vi "roboRIO v1.0 Write DIO.vi"(8 "error in (no error)":errorcluster, 9 "bool Value List":bool[](array[boolean]), 10 "Channel List":T3, 11 "myRIO Ref In":T1) -> (0 "error out":errorcluster, 3 "myRIO Ref Out":T1)   [LabVIEW 2021]
uses:
  <vilib>/myRIO/Common/Instrument Driver Framework/myRIO v1.0/DIO/typedefs/DIO Channels List.ctl
  <vilib>/myRIO/Common/Instrument Driver Framework/myRIO v1.0/DIO/typedefs/DIO Channels Enum.ctl
  <vilib>/myRIO/Common/Instrument Driver Framework/Utilities/typedefs/myRIO v1.0 Reference.ctl
  <vilib>/myRIO/Common/Instrument Driver Framework/Utilities/typedefs/Generic FPGA Reference.ctl
  <vilib>/myRIO/Common/Instrument Driver Framework/roboRIO v1.0/DIO/typedefs/roboRIO DIO FPGA Reference.ctl
  <vilib>/myRIO/Common/Instrument Driver Framework/roboRIO v1.0/DIO/typedefs/roboRIO DIO Bank Enum.ctl
  <vilib>/rvi/errors/niLvFpgaAdjustHostInterfaceError.vi
  <vilib>/rvi/interface/nirviReadWriteControl/nirviReadWriteControl.xnode
  <vilib>/rvi/interface/Simulation/niFpgaSimulationCallBeginRW.vi
  NiFpgaLv.dll
panel:
  # "This VI writes boolean values to a user specified a list of DIO channels on the myRIO v1.0 hardware. The value is input as a boolean value. Please see Block Diagram for details."
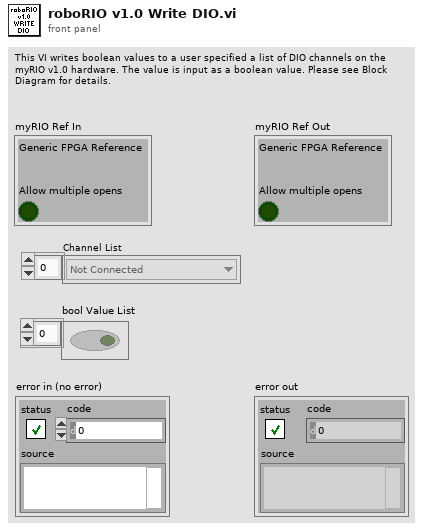
[diagram p1: front panel]
types:
  T1 = typedef "myRIO v1.0 Reference.ctl" = cluster{"Generic FPGA Reference":T2, "Allow multiple opens":bool}
  T2 = typedef "Generic FPGA Reference.ctl" = refnum<k20>
  T3 = typedef "DIO Channels List.ctl" = T4[]
  T4 = typedef "DIO Channels Enum.ctl" = enum16{"Not Connected", "C/DIO0", "C/DIO1", "C/DIO2", "C/DIO3", "C/DIO4", "C/DIO5", "C/DIO6", "C/DIO7", "A/DIO0", "A/DIO1", "A/DIO2", "A/DIO3", "A/DIO4", "A/DIO5", "A/DIO6", "A/DIO7", "A/DIO8", "A/DIO9", "A/DIO10", "A/DIO11", "A/DIO12", "A/DIO13", "A/DIO14", "A/DIO15", "A/DIO16", "A/DIO17", "A/DIO18", "A/DIO19", "B/DIO0", "B/DIO1", "B/DIO2", "B/DIO3", "B/DIO4", "B/DIO5", "B/DIO6", "B/DIO7", "B/DIO8", "B/DIO9", "B/DIO10", "B/DIO11", "B/DIO12", "B/DIO13", "B/DIO14", "B/DIO15", "B/DIO16", "B/DIO17", "B/DIO18", "B/DIO19", "LED0", "LED1", "LED2", "LED3", "Button0", "DIO/DIO0", "DIO/DIO1", "DIO/DIO2", "DIO/DIO3", "DIO/DIO4", "DIO/DIO5", "DIO/DIO6", "DIO/DIO7", "DIO/DIO8", "DIO/DIO9", "SPI/CS0", "SPI/CS1", "SPI/CS2", "SPI/CS3", "LED RADIO (Green)", "LED RADIO (Red)", "LED COMM (Green)", "LED COMM (Red)", "LED MODE (Green)", "LED MODE (Red)"}
  T5 = typedef "roboRIO DIO Bank Enum.ctl" = enum32{"None", "B/DIO7:0", "B/DIO15:8", "DIO/DIO7:0", "DIO/DIO9:8", "SPI/CS3:0", "LED", "Button0"}
  T6 = typedef "roboRIO DIO FPGA Reference.ctl" = refnum<k20>
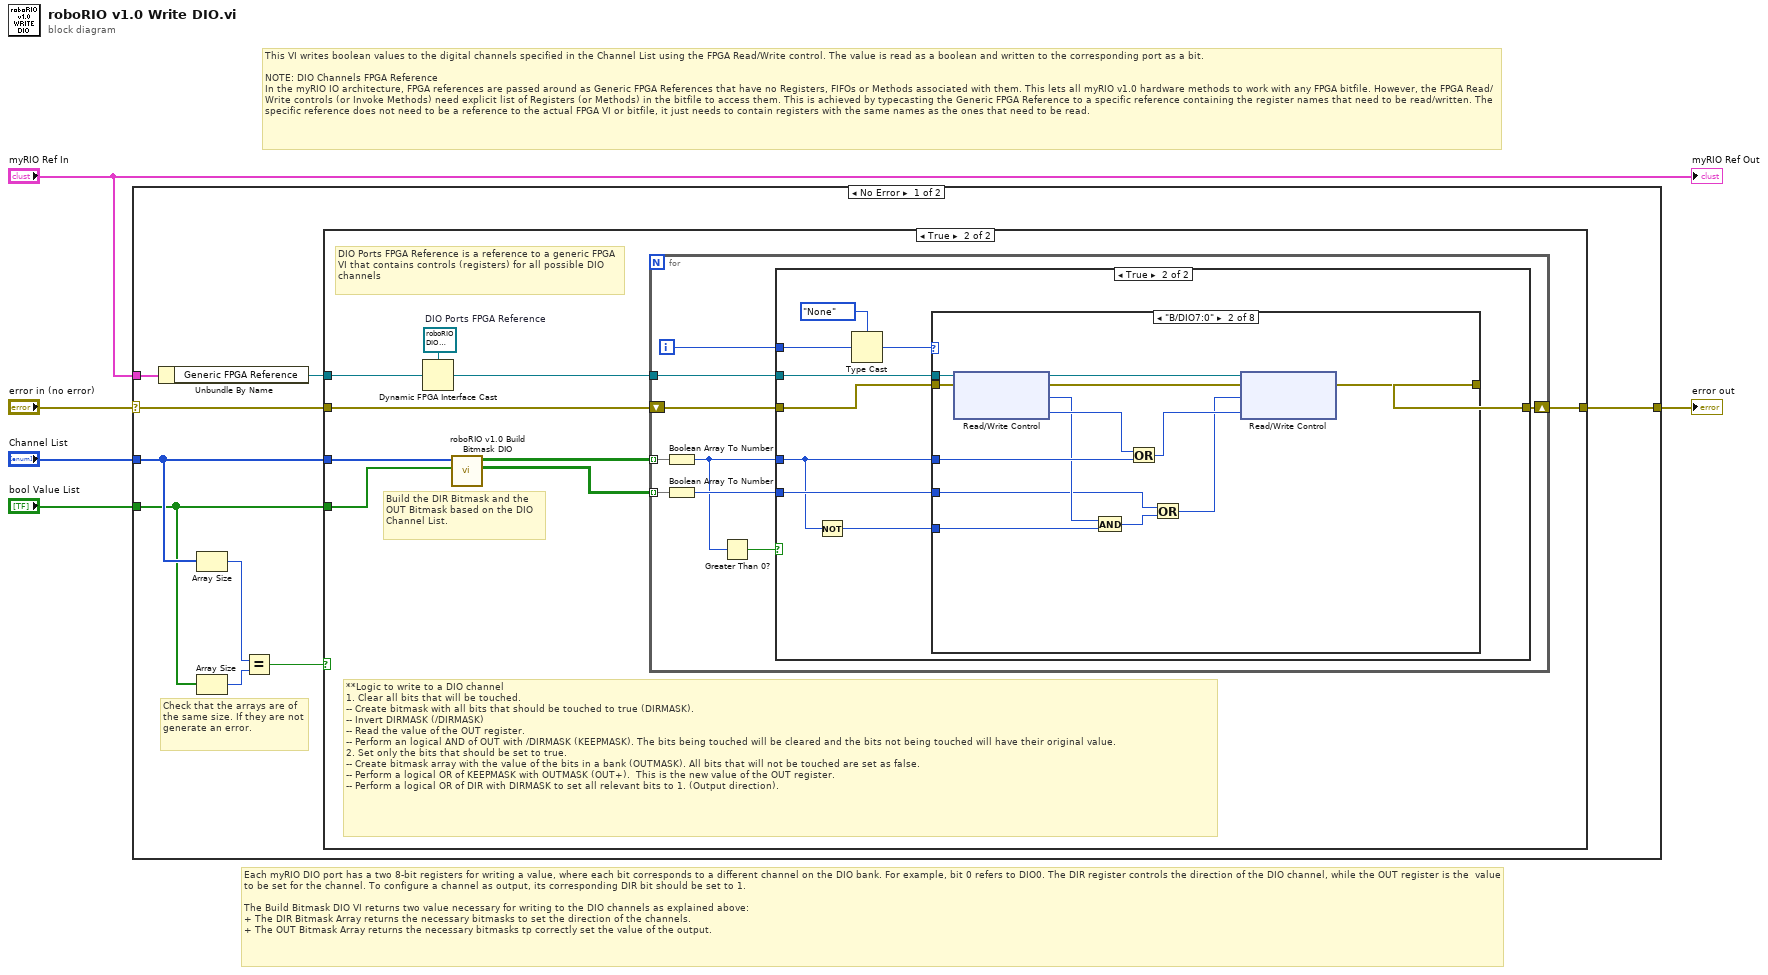
[diagram p0: block diagram]
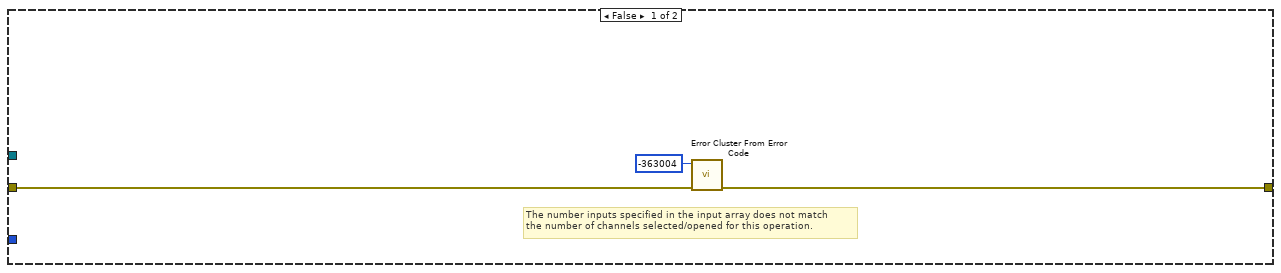
[diagram p2: hidden frame]
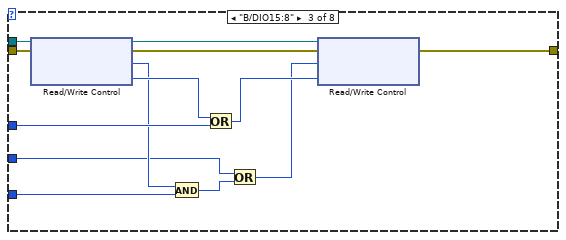
[diagram p5: hidden frame]
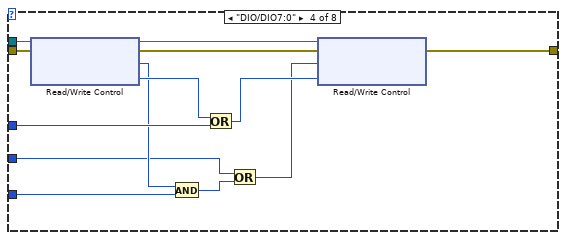
[diagram p6: hidden frame]
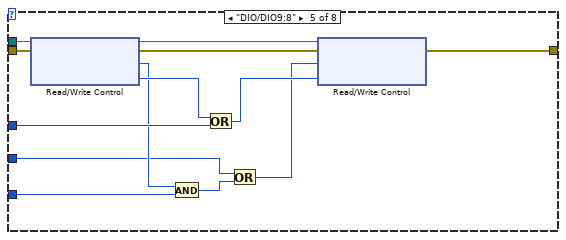
[diagram p7: hidden frame]
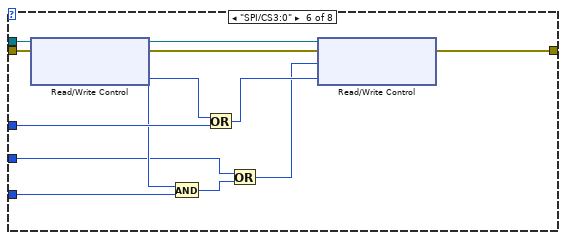
[diagram p8: hidden frame]
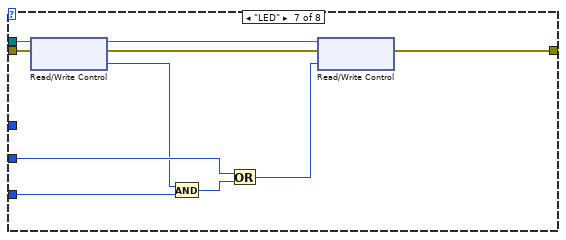
[diagram p9: hidden frame]
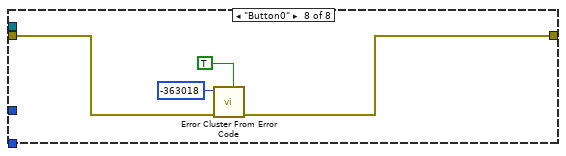
[diagram p10: hidden frame]
diagram:
  # "Each myRIO DIO port has a two 8-bit registers for writing a value, where each bit corresponds to a different channel on the DIO bank. For example, bit 0 refers to DIO0. The DIR register controls the direction of the DIO channel, while the OUT register is the  value to be set for the channel. To configure a channel as output, its corresponding DIR bit should be set to 1.\n\nThe Build Bitmask DIO VI returns two value necessary for writing to the DIO channels as explained above:\n+ The DIR Bitmask Array returns the necessary bitmasks to set the direction of the channels.\n+ The OUT Bitmask Array returns the necessary bitmasks tp correctly set the value of the output."
  # "This VI writes boolean values to the digital channels specified in the Channel List using the FPGA Read/Write control. The value is read as a boolean and written to the corresponding port as a bit. \n\nNOTE: DIO Channels FPGA Reference\nIn the myRIO IO architecture, FPGA references are passed around as Generic FPGA References that have no Registers, FIFOs or Methods associated with them. This lets all myRIO v1.0 hardware methods to work with any FPGA bitfile. However, the FPGA Read/Write controls (or Invoke Methods) need explicit list of Registers (or Methods) in the bitfile to access them. This is achieved by typecasting the Generic FPGA Reference to a specific reference containing the register names that need to be read/written. The specific reference does not need to be a reference to the actual FPGA VI or bitfile, it just needs to contain registers with the same names as the ones that need to be read."
  n1 = case shown="No Error" "error in (no error)" {
    selector: "error in (no error)" -> [w7 w126]
    tunnel: "myRIO Ref In" -> [w14 _]
    tunnel: [w13 w126] -> w4
    tunnel: "Channel List" -> [w10 _]
    tunnel: "bool Value List" -> [w9 _]
    frame No Error {
      # "Check that the arrays are of the same size. If they are not generate an error."
      n2 = Unbundle By Name(w14) -> ("Generic FPGA Reference"=w6:T2)
      n3 = Array Size(array=w10) -> (size(s)=w12:i32)
      n4 = Array Size(array=w9) -> (size(s)=w11:i32)
      n5 = Equal?(x=w12, y=w11) -> (x = y?=w8:bool)
      n6 = case shown="True" w8 {
        tunnel: w10 -> [_ w26]
        tunnel: w9 -> [_ w25]
        tunnel: w6 -> [_ w23]
        tunnel: w7 -> [w16 w21]
        tunnel: [w15 w20] -> w13
        frame False {
          # "The number inputs specified in the input array does not match\nthe number of channels selected/opened for this operation."
          n7 = call <vilib>:"Error Cluster From Error Code.vi"("error in (no error)"=w16, "error code (0)"=-363004) -> ("error out"=w15:errorcluster)  [unwired: 7 in]
        }
        frame True {
          w24 = T6 refnum  # DIO Ports FPGA Reference
          # "DIO Ports FPGA Reference is a reference to a generic FPGA VI that contains controls (registers) for all possible DIO channels"
          # "Build the DIR Bitmask and the OUT Bitmask based on the DIO Channel List."
          # "**Logic to write to a DIO channel\n1. Clear all bits that will be touched.\n-- Create bitmask with all bits that should be touched to true (DIRMASK).\n-- Invert DIRMASK (/DIRMASK)\n-- Read the value of the OUT register.\n-- Perform an logical AND of OUT with /DIRMASK (KEEPMASK). The bits being touched will be cleared and the bits not being touched will have their original value.\n2. Set only the bits that should be set to true.\n-- Create bitmask array with the value of the bits in a bank (OUTMASK). All bits that will not be touched are set as false.\n-- Perform a logical OR of KEEPMASK with OUTMASK (OUT+).  This is the new value of the OUT register.\n-- Perform a logical OR of DIR with DIRMASK to set all relevant bits to 1. (Output direction)."
          n8 = Dynamic FPGA Interface Cast(Session In=w24, Type=w23) -> (Session Out=w22:T6)
          n9 = call <vilib>:"roboRIO v1.0 Build Bitmask DIO.vi"("bool Value List In"=w25, "Channel List"=w26) -> ("OUT Bitmask Array"=w18:bool[][], "DIR Bitmask Array"=w19:bool[][])  [unwired: 7 in, 1 out]
          n10 = for {
            tunnel: w22 -> [w35]
            tunnel: w19 -> [w32] mode=indexing
            shift-right: [w30] -> w20
            shift-left: w21 -> [w34]
            tunnel: w18 -> [w29] mode=indexing
            i -> [w33]
            n11 = Boolean Array To Number(Boolean array=w32) -> (number=w27:u8)
            n12 = Boolean Array To Number(Boolean array=w29) -> (number=w31:u8)
            n13 = Greater Than 0?(x=w27) -> (x > 0?=w28:bool)
            n14 = case shown="True" w28 {
              tunnel: w35 -> [_ w45]
              tunnel: w34 -> [w36 w44]
              tunnel: w33 -> [_ w42]
              tunnel: w31 -> [_ w40]
              tunnel: w27 -> [_ w39]
              tunnel: [w36 w37] -> w30
              frame False {
              }
              frame True {
                n15 = Not(x=w39) -> (.not. x?=w38:u8)
                n16 = Type Cast(type=roboRIO_DIO_Bank_Enum."None" ("DIO Bank Enum"), x=w42) -> (*(type *) &x=w41:T5)
                n17 = case shown="\"B/DIO7:0\"" w41 {
                  tunnel: w45 -> [_ w59 w72 w85 w98 w111 w121 _]
                  tunnel: w44 -> [w46 w58 w71 w84 w97 w110 w120 w125]
                  tunnel: w39 -> [_ w56 w69 w82 w95 w108 _ _]
                  tunnel: w40 -> [_ w52 w65 w78 w91 w104 w118 _]
                  tunnel: w38 -> [_ w53 w66 w79 w92 w105 w119 _]
                  tunnel: [w46 w47 w60 w73 w86 w99 w114 w124] -> w37
                  frame "None", Default {
                  }
                  frame "B/DIO7:0" {
                    n18 = xnode "Read/Write Control"("FPGA VI Reference In"=w59, "error in"=w58) -> ("FPGA VI Reference Out"=w49:T6, "error out"=w48:errorcluster, "DIO.B_7:0.OUT"=w54:u8, "DIO.B_7:0.DIR"=w57:u8)
                    n19 = And(x=w54, y=w53) -> (x .and. y?=w51:u8)
                    n20 = Or(x=w57, y=w56) -> (x .or. y?=w55:u8)
                    n21 = Or(x=w52, y=w51) -> (x .or. y?=w50:u8)
                    n22 = xnode "Read/Write Control"("FPGA VI Reference In"=w49, "error in"=w48, "DIO.B_7:0.OUT"=w50, "DIO.B_7:0.DIR"=w55) -> ("error out"=w47:errorcluster)  [unwired: 1 out]
                  }
                  frame "B/DIO15:8" {
                    n23 = xnode "Read/Write Control"("FPGA VI Reference In"=w72, "error in"=w71) -> ("FPGA VI Reference Out"=w62:T6, "error out"=w61:errorcluster, "DIO.B_15:8.OUT"=w67:u8, "DIO.B_15:8.DIR"=w70:u8)
                    n24 = And(x=w67, y=w66) -> (x .and. y?=w64:u8)
                    n25 = Or(x=w70, y=w69) -> (x .or. y?=w68:u8)
                    n26 = Or(x=w65, y=w64) -> (x .or. y?=w63:u8)
                    n27 = xnode "Read/Write Control"("FPGA VI Reference In"=w62, "error in"=w61, "DIO.B_15:8.OUT"=w63, "DIO.B_15:8.DIR"=w68) -> ("error out"=w60:errorcluster)  [unwired: 1 out]
                  }
                  frame "DIO/DIO7:0" {
                    n28 = xnode "Read/Write Control"("FPGA VI Reference In"=w85, "error in"=w84) -> ("FPGA VI Reference Out"=w75:T6, "error out"=w74:errorcluster, "DIO.DIO_7:0.OUT"=w80:u8, "DIO.DIO_7:0.DIR"=w83:u8)
                    n29 = And(x=w80, y=w79) -> (x .and. y?=w77:u8)
                    n30 = Or(x=w83, y=w82) -> (x .or. y?=w81:u8)
                    n31 = Or(x=w78, y=w77) -> (x .or. y?=w76:u8)
                    n32 = xnode "Read/Write Control"("FPGA VI Reference In"=w75, "error in"=w74, "DIO.DIO_7:0.OUT"=w76, "DIO.DIO_7:0.DIR"=w81) -> ("error out"=w73:errorcluster)  [unwired: 1 out]
                  }
                  frame "DIO/DIO9:8" {
                    n33 = xnode "Read/Write Control"("FPGA VI Reference In"=w98, "error in"=w97) -> ("FPGA VI Reference Out"=w88:T6, "error out"=w87:errorcluster, "DIO.DIO_9:8.OUT"=w93:u8, "DIO.DIO_9:8.DIR"=w96:u8)
                    n34 = And(x=w93, y=w92) -> (x .and. y?=w90:u8)
                    n35 = Or(x=w96, y=w95) -> (x .or. y?=w94:u8)
                    n36 = Or(x=w91, y=w90) -> (x .or. y?=w89:u8)
                    n37 = xnode "Read/Write Control"("FPGA VI Reference In"=w88, "error in"=w87, "DIO.DIO_9:8.OUT"=w89, "DIO.DIO_9:8.DIR"=w94) -> ("error out"=w86:errorcluster)  [unwired: 1 out]
                  }
                  frame "SPI/CS3:0" {
                    n38 = xnode "Read/Write Control"("FPGA VI Reference In"=w111, "error in"=w110) -> ("FPGA VI Reference Out"=w101:T6, "error out"=w100:errorcluster, "DIO.SPI_CS3:0.OUT"=w106:u8, "DIO.SPI_CS3:0.DIR"=w109:u8)
                    n39 = And(x=w106, y=w105) -> (x .and. y?=w103:u8)
                    n40 = Or(x=w109, y=w108) -> (x .or. y?=w107:u8)
                    n41 = Or(x=w104, y=w103) -> (x .or. y?=w102:u8)
                    n42 = xnode "Read/Write Control"("FPGA VI Reference In"=w101, "error in"=w100, "DIO.SPI_CS3:0.OUT"=w102, "DIO.SPI_CS3:0.DIR"=w107) -> ("error out"=w99:errorcluster)  [unwired: 1 out]
                  }
                  frame "LED" {
                    n43 = xnode "Read/Write Control"("FPGA VI Reference In"=w121, "error in"=w120) -> ("FPGA VI Reference Out"=w116:T6, "error out"=w115:errorcluster, "DO.LED 5:0"=w113:u8)
                    n44 = And(x=w113, y=w119) -> (x .and. y?=w117:u8)
                    n45 = Or(x=w118, y=w117) -> (x .or. y?=w112:u8)
                    n46 = xnode "Read/Write Control"("FPGA VI Reference In"=w116, "error in"=w115, "DO.LED 5:0"=w112) -> ("error out"=w114:errorcluster)  [unwired: 1 out]
                  }
                  frame "Button0" {
                    n47 = call <vilib>:"Error Cluster From Error Code.vi"("is warning? (False)"=TRUE, "error in (no error)"=w125, "error code (0)"=-363018) -> ("error out"=w124:errorcluster)  [unwired: 6 in]
                  }
                }
              }
            }
          }
        }
      }
    }
    frame Error {
    }
  }
  "error out" <- w4
  "myRIO Ref Out" <- "myRIO Ref In"
